vi "Analysis.vi"(6 "Functions":T3(ring)=enum."Measurement", 7 "error in":errorcluster, 8 "Scan/Meas Parameters":T2={"Pixel Dwell Time (s)"=0.0001, "Pixel Size"=200.0, "X Min (V)"=-7.5, "X Max (V)"=7.5, "Y Min (V)"=-7.5, "Y Max (V)"=7.5, "XY Factor (1/V)"=0.2}, 9 "Global Parameters":T1={"DC AI Min (V)"=0.0015, "DC AI Max (V)"=0.06, "Mixer AI Min (V)"=-0.3, "Mixer AI Max (V)"=0.3, "Bias AO Min (V)"=-1.0, "Bias AO Max (V)"=7.0, "Scan AO Min (V)"=-10.0, "Scan AO Max (V)"=10.0, "Fast Samp Freq (Hz)"=2500000.0, "Slow Samp Freq (Hz)"=250000.0}, 10 "DC AI Channel Data":dbl[](array[numeric]) format="%0.2f", 11 "Mixer AI Channels Data":dbl[][](array[numeric]) format="%0.2f") -> (0 "AI Mix4 Data":dbl[](array[numeric]), 1 "AI Mix3 Data":dbl[](array[numeric]), 2 "AI Mix2 Data":dbl[](array[numeric]), 3 "AI Mix1 Data":dbl[](array[numeric]), 4 "AI DC Data":dbl[](array[numeric]), 5 "error out":errorcluster)   [LabVIEW 2018]
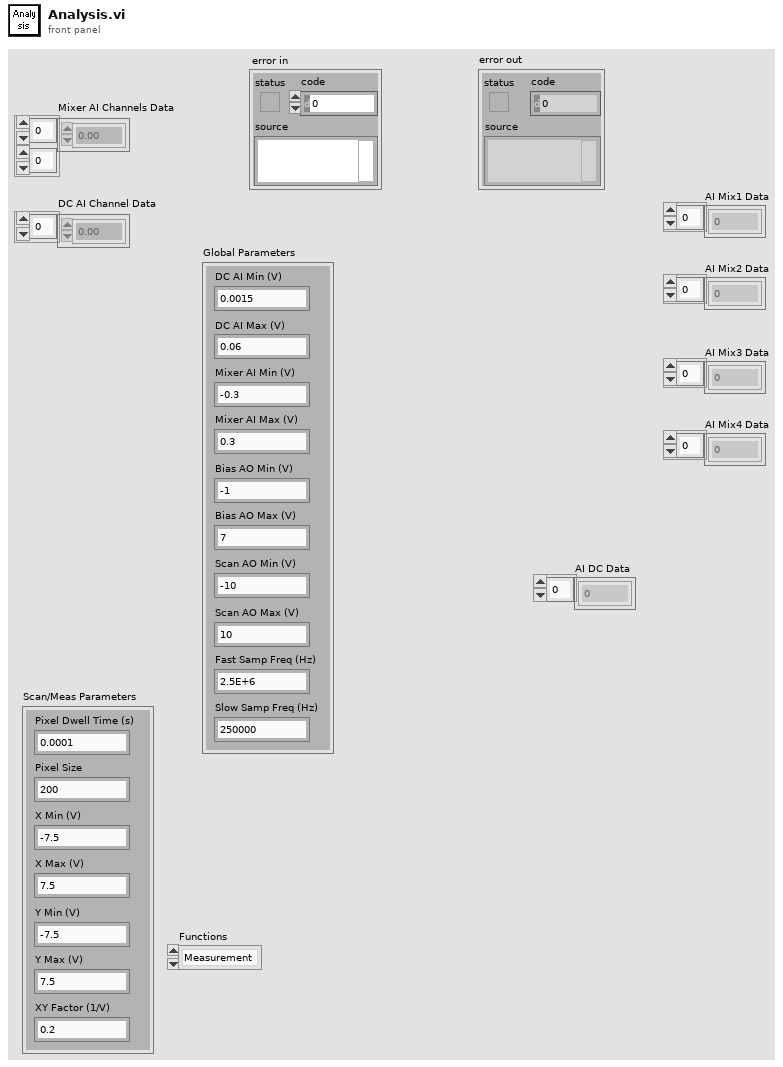
[diagram p1: front panel]
types:
  T1 = cluster{"DC AI Min (V)":dbl, "DC AI Max (V)":dbl, "Mixer AI Min (V)":dbl, "Mixer AI Max (V)":dbl, "Bias AO Min (V)":dbl, "Bias AO Max (V)":dbl, "Scan AO Min (V)":dbl, "Scan AO Max (V)":dbl, "Fast Samp Freq (Hz)":dbl, "Slow Samp Freq (Hz)":dbl}
  T2 = cluster{"Pixel Dwell Time (s)":dbl, "Pixel Size":dbl, "X Min (V)":dbl, "X Max (V)":dbl, "Y Min (V)":dbl, "Y Max (V)":dbl, "XY Factor (1/V)":dbl}
  T3 = enum32{"Calibration", "Fast Scan", "Measurement"}
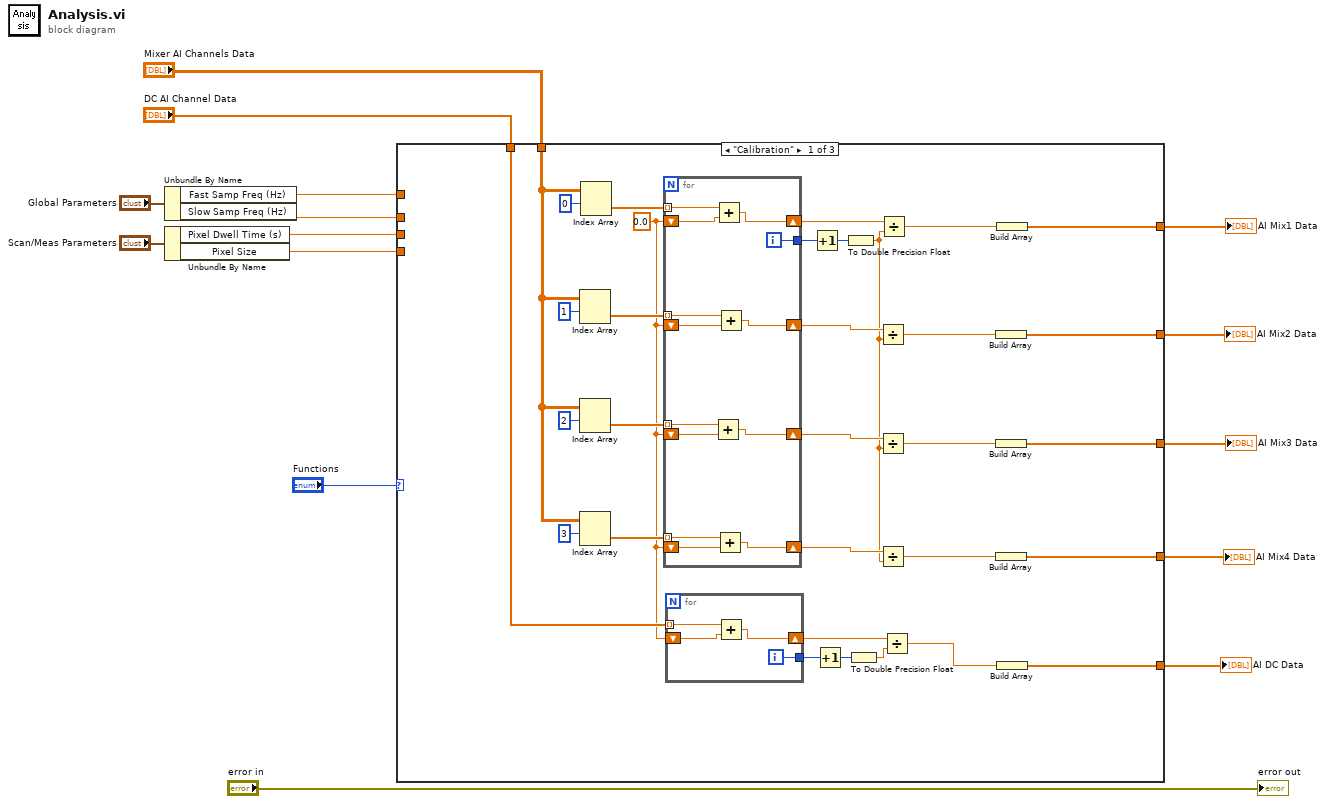
[diagram p0: block diagram]
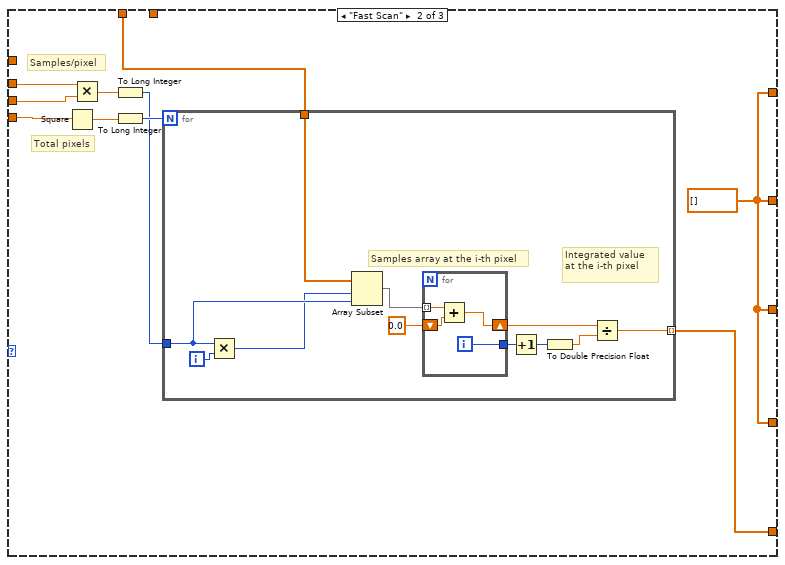
[diagram p2: hidden frame]
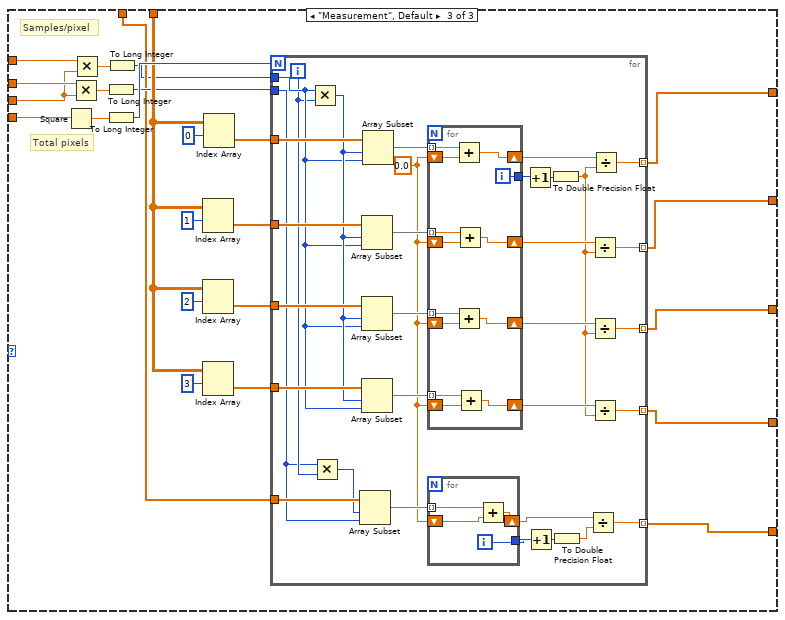
[diagram p3: hidden frame]
diagram:
  n1 = Unbundle By Name("Global Parameters") -> ("Fast Samp Freq (Hz)"=w3:dbl, "Slow Samp Freq (Hz)"=w13:dbl)
  n2 = Unbundle By Name("Scan/Meas Parameters") -> ("Pixel Dwell Time (s)"=w12:dbl, "Pixel Size"=w11:dbl)
  n3 = case shown="\"Calibration\"" "Functions" {
    tunnel: w13 -> [_ w72 w112]
    tunnel: w12 -> [_ w71 w92]
    tunnel: w11 -> [_ w70 w111]
    tunnel: "Mixer AI Channels Data" -> [w27 _ w99]
    tunnel: [w45 w68 w110] -> w10
    tunnel: [w24 w69 w104] -> w8
    tunnel: [w36 w68 w107] -> w7
    tunnel: [w35 w68 w106] -> w6
    tunnel: [w34 w68 w105] -> w5
    tunnel: "DC AI Channel Data" -> [w21 w65 w94]
    tunnel: w3 -> [_ _ w91]
    frame "Calibration" {
      w16 = 0.0
      n4 = Index Array(array=w27, index (row)=1) -> (element=w33:dbl[])  [unwired: 1 in]
      n5 = Index Array(array=w27, index (row)=2) -> (element=w32:dbl[])  [unwired: 1 in]
      n6 = Index Array(array=w27, index (row)=3) -> (element=w31:dbl[])  [unwired: 1 in]
      n7 = Index Array(array=w27, index (row)=0) -> (element=w43:dbl[])  [unwired: 1 in]
      n8 = for {
        tunnel: w43 -> [w64] mode=indexing
        shift-right: [w62] -> w47
        shift-left: w16 -> [w63]
        tunnel: [w61] -> w23
        tunnel: w33 -> [w60] mode=indexing
        tunnel: w32 -> [w59] mode=indexing
        tunnel: w31 -> [w58] mode=indexing
        shift-right: [w54] -> w30
        shift-left: w16 -> [w57]
        shift-right: [w53] -> w29
        shift-left: w16 -> [w56]
        shift-right: [w52] -> w28
        shift-left: w16 -> [w55]
        i -> [w61]
        n9 = Add(x=w59, y=w56) -> (x+y=w53:dbl)
        n10 = Add(x=w64, y=w63) -> (x+y=w62:dbl)
        n11 = Add(x=w58, y=w55) -> (x+y=w52:dbl)
        n12 = Add(x=w60, y=w57) -> (x+y=w54:dbl)
      }
      n13 = for {
        tunnel: w21 -> [w51] mode=indexing
        shift-right: [w49] -> w20
        shift-left: w16 -> [w50]
        tunnel: [w48] -> w18
        i -> [w48]
        n14 = Add(x=w51, y=w50) -> (x+y=w49:dbl)
      }
      n15 = Increment(x=w23) -> (x+1=w22:i32)
      n16 = Increment(x=w18) -> (x+1=w19:i32)
      n17 = To Double Precision Float(number=w22) -> (double precision float=w25:dbl)
      n18 = To Double Precision Float(number=w19) -> (double precision float=w17:dbl)
      n19 = Divide(x=w30, y=w25) -> (x/y=w42:dbl)
      n20 = Divide(x=w29, y=w25) -> (x/y=w40:dbl)
      n21 = Divide(x=w28, y=w25) -> (x/y=w38:dbl)
      n22 = Divide(x=w47, y=w25) -> (x/y=w46:dbl)
      n23 = Divide(x=w20, y=w17) -> (x/y=w26:dbl)
      n24 = Build Array(w42) -> (w36:dbl[])
      n25 = Build Array(w40) -> (w35:dbl[])
      n26 = Build Array(w38) -> (w34:dbl[])
      n27 = Build Array(w46) -> (w45:dbl[])
      n28 = Build Array(w26) -> (w24:dbl[])
    }
    frame "Fast Scan" {
      w68 = dbl[] []
      # "Total pixels"
      # "Samples/pixel"
      n29 = Square(x=w70) -> (x^2=w73:dbl)
      n30 = Multiply(x=w72, y=w71) -> (x*y=w67:dbl)
      n31 = To Long Integer(number=w67) -> (32bit integer=w66:i32)
      n32 = To Long Integer(number=w73) -> (32bit integer=w74:i32)
      n33 = for {
        N: w74 -> [_]
        tunnel: w65 -> [w85]
        tunnel: w66 -> [w83]
        tunnel: [w79] -> w69 mode=indexing
        i -> [w84]
        # "Integrated value at the i-th pixel"
        # "Samples array at the i-th pixel"
        n34 = Multiply(x=w83, y=w84) -> (x*y=w78:i32)
        n35 = Array Subset(array=w85, index=w78, length=w83) -> (w80:dbl[])
        n36 = for {
          tunnel: w80 -> [w89] mode=indexing
          shift-right: [w87] -> w81
          shift-left: 0.0 -> [w88]
          tunnel: [w86] -> w77
          i -> [w86]
          n37 = Add(x=w89, y=w88) -> (x+y=w87:dbl)
        }
        n38 = Increment(x=w77) -> (x+1=w76:i32)
        n39 = To Double Precision Float(number=w76) -> (double precision float=w75:dbl)
        n40 = Divide(x=w81, y=w75) -> (x/y=w79:dbl)
      }
    }
    frame "Measurement", Default {
      # "Total pixels"
      # "Samples/pixel"
      n41 = Square(x=w111) -> (x^2=w114:dbl)
      n42 = Multiply(x=w112, y=w92) -> (x*y=w96:dbl)
      n43 = Multiply(x=w91, y=w92) -> (x*y=w93:dbl)
      n44 = To Long Integer(number=w96) -> (32bit integer=w95:i32)
      n45 = To Long Integer(number=w114) -> (32bit integer=w113:i32)
      n46 = To Long Integer(number=w93) -> (32bit integer=w90:i32)
      n47 = Index Array(array=w99, index (row)=1) -> (element=w102:dbl[])  [unwired: 1 in]
      n48 = Index Array(array=w99, index (row)=2) -> (element=w98:dbl[])  [unwired: 1 in]
      n49 = Index Array(array=w99, index (row)=3) -> (element=w97:dbl[])  [unwired: 1 in]
      n50 = Index Array(array=w99, index (row)=0) -> (element=w103:dbl[])  [unwired: 1 in]
      n51 = for {
        N: w113 -> [_]
        tunnel: w95 -> [w116]
        tunnel: [w144] -> w110 mode=indexing
        tunnel: [w143] -> w107 mode=indexing
        tunnel: [w142] -> w106 mode=indexing
        tunnel: [w141] -> w105 mode=indexing
        tunnel: [w140] -> w104 mode=indexing
        tunnel: w103 -> [w139]
        tunnel: w102 -> [w138]
        tunnel: w98 -> [w137]
        tunnel: w97 -> [w136]
        tunnel: w94 -> [w135]
        tunnel: w90 -> [w118]
        i -> [w117]
        w123 = 0.0
        n52 = Multiply(x=w118, y=w117) -> (x*y=w134:i32)
        n53 = Multiply(x=w116, y=w117) -> (x*y=w115:i32)
        n54 = Array Subset(array=w135, index=w115, length=w116) -> (w124:dbl[])
        n55 = Array Subset(array=w138, index=w134, length=w118) -> (w133:dbl[])
        n56 = Array Subset(array=w137, index=w134, length=w118) -> (w132:dbl[])
        n57 = Array Subset(array=w136, index=w134, length=w118) -> (w131:dbl[])
        n58 = Array Subset(array=w139, index=w134, length=w118) -> (w145:dbl[])
        n59 = for {
          tunnel: w145 -> [w160] mode=indexing
          shift-right: [w162] -> w146
          shift-left: w123 -> [w163]
          tunnel: [w161] -> w126
          tunnel: w133 -> [w159] mode=indexing
          tunnel: w132 -> [w158] mode=indexing
          tunnel: w131 -> [w157] mode=indexing
          shift-right: [w153] -> w130
          shift-left: w123 -> [w156]
          shift-right: [w152] -> w129
          shift-left: w123 -> [w155]
          shift-right: [w151] -> w128
          shift-left: w123 -> [w154]
          i -> [w161]
          n60 = Add(x=w160, y=w163) -> (x+y=w162:dbl)
          n61 = Add(x=w158, y=w155) -> (x+y=w152:dbl)
          n62 = Add(x=w159, y=w156) -> (x+y=w153:dbl)
          n63 = Add(x=w157, y=w154) -> (x+y=w151:dbl)
        }
        n64 = for {
          tunnel: w124 -> [w150] mode=indexing
          shift-right: [w148] -> w122
          shift-left: w123 -> [w149]
          tunnel: [w147] -> w120
          i -> [w147]
          n65 = Add(x=w150, y=w149) -> (x+y=w148:dbl)
        }
        n66 = Increment(x=w126) -> (x+1=w125:i32)
        n67 = Increment(x=w120) -> (x+1=w121:i32)
        n68 = To Double Precision Float(number=w125) -> (double precision float=w127:dbl)
        n69 = To Double Precision Float(number=w121) -> (double precision float=w119:dbl)
        n70 = Divide(x=w122, y=w119) -> (x/y=w140:dbl)
        n71 = Divide(x=w130, y=w127) -> (x/y=w143:dbl)
        n72 = Divide(x=w129, y=w127) -> (x/y=w142:dbl)
        n73 = Divide(x=w128, y=w127) -> (x/y=w141:dbl)
        n74 = Divide(x=w146, y=w127) -> (x/y=w144:dbl)
      }
    }
  }
  "AI Mix1 Data" <- w10
  "AI DC Data" <- w8
  "AI Mix2 Data" <- w7
  "AI Mix3 Data" <- w6
  "AI Mix4 Data" <- w5
  "error out" <- "error in"
